vi "UI_Initialize_Panel.vi"(8 "error in (no error)":errorcluster caption="entrée d'erreur (pas d'erreur)", 10 "QMH UI Cluster":T1) -> (0 "error out":errorcluster caption="sortie d'erreur", 2 "QMH UI Cluster":T1)   [LabVIEW 2015]
uses:
  controls/QMH_UI_Cluster.ctl
  controls/QMH_UI_References.ctl
  controls/QMH_UI_Report.ctl
  controls/QMH_UI_Command.ctl
  controls/QMH_ICR_Command.ctl
  controls/QMH_Status.ctl
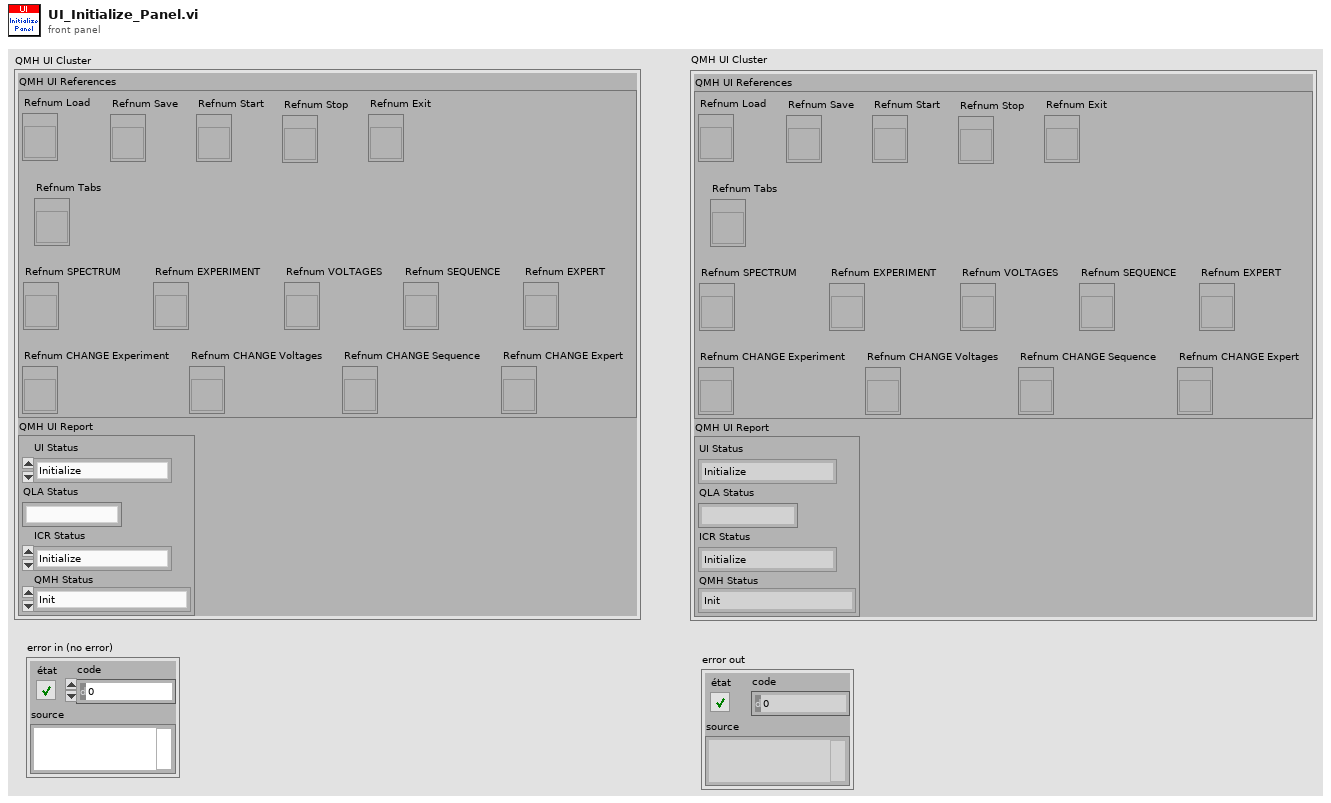
[diagram p1: front panel]
types:
  T1 = typedef "QMH_UI_Cluster.ctl" = cluster{"QMH UI References":T2, "QMH UI Report":T3}
  T2 = typedef "QMH_UI_References.ctl" = cluster{"Refnum Load":refnum<vi>, "Refnum Save":refnum<vi>, "Refnum Start":refnum<vi>, "Refnum Stop":refnum<vi>, "Refnum Exit":refnum<vi>, "Refnum Tabs":refnum<vi>, "Refnum SPECTRUM":refnum<vi>, "Refnum EXPERIMENT":refnum<vi>, "Refnum VOLTAGES":refnum<vi>, "Refnum SEQUENCE":refnum<vi>, "Refnum EXPERT":refnum<vi>, "Refnum CHANGE Experiment":refnum<vi>, "Refnum CHANGE Voltages":refnum<vi>, "Refnum CHANGE Sequence":refnum<vi>, "Refnum CHANGE Expert":refnum<vi>}
  T3 = typedef "QMH_UI_Report.ctl" = cluster{"UI Status":T4, "QLA Status":string, "ICR Status":T5, "QMH Status":T6}
  T4 = typedef "QMH_UI_Command.ctl" = enum16{"Initialize", "UI Load", "UI Save", "UI Change Experiment", "UI Change Voltages", "UI Change Sequence", "UI Change Expert", "Ready to Start", "UI Start", "UI Stop", "UI Exit", "Update Report", "Update ICR Report"}
  T5 = typedef "QMH_ICR_Command.ctl" = enum16{"Initialize", "Hardware Setup", "Waiting for Trigger", "Sequence Started", "Sequence Finished", "Writing Data", "Hardware Reset", "Exit"}
  T6 = typedef "QMH_Status.ctl" = enum16{"Init", "Loading", "Setup", "Ready to Start", "Started", "Idle"}
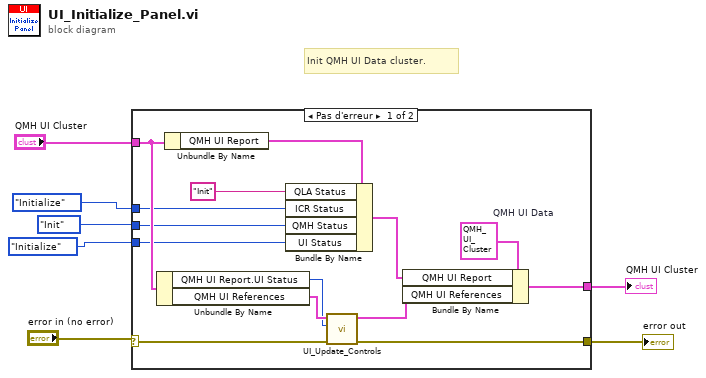
[diagram p0: block diagram]
diagram:
  # "Init QMH UI Data cluster."
  n1 = case shown="Pas d'erreur" "error in (no error)" {
    selector: "error in (no error)" -> [w19 w22]
    tunnel: "QMH UI Cluster" -> [w14 _]
    tunnel: [w18 w22] -> w5
    tunnel: QMH_Status."Init" ("QMH Status") -> [w11 _]
    tunnel: [w16 _] -> w3
    tunnel: QMH_ICR_Command."Initialize" ("ICR Status") -> [w10 _]
    tunnel: QMH_UI_Command."Initialize" ("UI Status") -> [w8 _]
    frame No Error {
      w21 = T1 {"QMH UI References"={"Refnum Load"=refnum, "Refnum Save"=refnum, "Refnum Start"=refnum, "Refnum Stop"=refnum, "Refnum Exit"=refnum, "Refnum Tabs"=refnum, "Refnum SPECTRUM"=refnum, "Refnum EXPERIMENT"=refnum, "Refnum VOLTAGES"=refnum, "Refnum SEQUENCE"=refnum, "Refnum EXPERT"=refnum, "Refnum CHANGE Experiment"=refnum, "Refnum CHANGE Voltages"=refnum, "Refnum CHANGE Sequence"=refnum, "Refnum CHANGE Expert"=refnum}, "QMH UI Report"={"UI Status"=enum."Initialize", "QLA Status"="", "ICR Status"=enum."Initialize", "QMH Status"=enum."Init"}}  # QMH UI Data
      n2 = Unbundle By Name(w14) -> ("QMH UI Report.UI Status"=w12:T4, "QMH UI References"=w13:T2)
      n3 = Unbundle By Name(w14) -> ("QMH UI Report"=w15:T3)
      n4 = Bundle By Name(cluster=w15, "QLA Status"="Init", "ICR Status"=w10, "QMH Status"=w11, "UI Status"=w8) -> (w20:T3)
      n5 = call "UI_Update_Controls.vi"("error in (no error)"=w19, "UI Status"=w12, "QMH UI References"=w13) -> ("error out"=w18:errorcluster, "QMH UI References"=w17:T2)  [unwired: 7 in]
      n6 = Bundle By Name(cluster=w21, "QMH UI Report"=w20, "QMH UI References"=w17) -> (w16:T1)
    }
    frame Error {
    }
  }
  "QMH UI Cluster" <- w3
  "error out" <- w5
